vi "View-camera-settings-with-dialog.vi"(8 "error in (no error)":errorcluster, 10 "UI ref. in":refnum<data-value>, 11 "Data ref. in":refnum<data-value>) -> (0 "error out":errorcluster, 3 "Data ref.":refnum<data-value>)   [LabVIEW 2013, in "CameraVision.lvlib" / "CV-Main.lvclass"]
uses:
  CV-Main.lvclass
  UI/CV-UI.lvclass
  CV-Main.lvclass/CV-Main.ctl
  Configuration/CV-Configuration.lvclass/CV-Configuration.ctl
  UI/CV-UI.lvclass/CV-UI.ctl
  Hardware/Camera/Camera.lvclass
  Read Config params.vi
  Configuration/Read Camera array.vi
  Configuration/Read Camport array.vi
  Configuration/Read Framegrabber board.vi
  UI/Read Camera.vi
  Configuration/CV-Configuration.lvclass
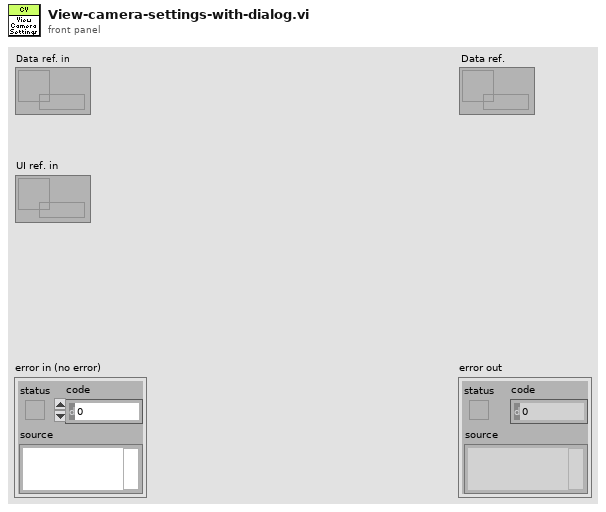
[diagram p1: front panel]
types:
  T1 = typedef "CameraVision.lvlib/CV-UI.lvclass/Camera-selector.ctl" = enum16{"Camera 1", "Camera 2"}
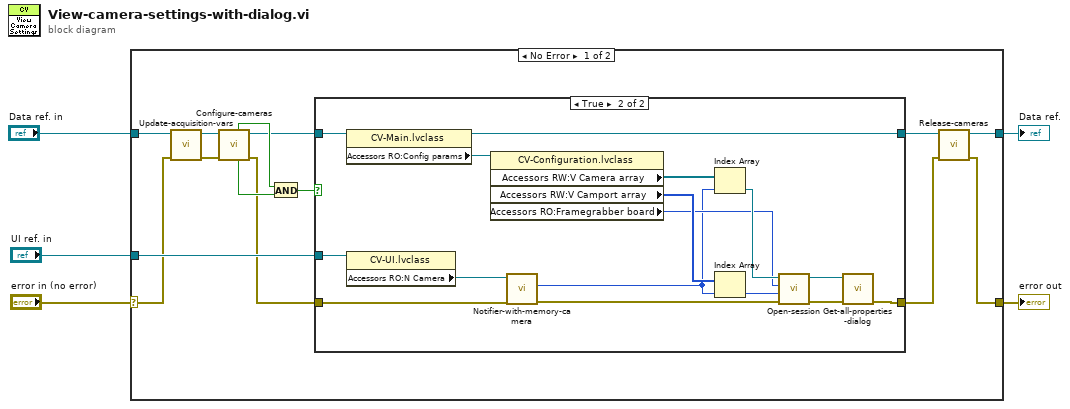
[diagram p0: block diagram]
diagram:
  n1 = case shown="No Error" "error in (no error)" {
    selector: "error in (no error)" -> [w10 w39]
    tunnel: [w9 w39] -> w4
    tunnel: [w6 w38] -> w2
    tunnel: "Data ref. in" -> [w14 w38]
    tunnel: "UI ref. in" -> [w19 _]
    frame No Error {
      n2 = call "Update-acquisition-vars.vi"("error in"=w10, "Data ref. in"=w14) -> ("error IO"=w16:errorcluster, "Data ref."=w15:refnum<data-value>)  [unwired: 6 in, 2 out]
      n3 = call "Configure-cameras.vi"("error in"=w16, "Data ref. in"=w15) -> ("error IO"=w11:errorcluster, "Data ref."=w13:refnum<data-value>, "Initialized?"=w18:bool, "Succes?"=w17:bool)  [unwired: 6 in]
      n4 = And(x=w17, y=w18) -> (x .and. y?=w12:bool)
      n5 = case shown="True" w12 {
        tunnel: [w21 w37] -> w7
        tunnel: w19 -> [_ w35]
        tunnel: w11 -> [w20 w32]
        tunnel: [w20 w24] -> w8
        tunnel: w13 -> [w21 w22]
        frame False {
        }
        frame True {
          n6 = property class="CV-Main.lvclass"(reference=w22) -> (reference out=w37:refnum<data-value>, "Accessors RO:Config params"=w36:refnum<data-value>)  [unwired: 1 in, 1 out]
          n7 = property class="CV-UI.lvclass"(reference=w35) -> ("Accessors RO:N Camera"=w34:refnum<notifier>)  [unwired: 1 in, 2 out]
          n8 = property class="CV-Configuration.lvclass"(reference=w36) -> ("Accessors RW:V Camera array"=w33:refnum<class "Camera.lvclass">[], "Accessors RW:V Camport array"=w27:u32[], "Accessors RO:Framegrabber board"=w26:i32)  [unwired: 1 in, 2 out]
          n9 = call "Notifier-with-memory-camera.vi"("error in"=w32, "Notifier in"=w34) -> ("error IO"=w29:errorcluster, "Notification"=w23:T1)  [unwired: 8 in]
          n10 = Index Array(array=w33, index=w23) -> (element=w30:refnum<class "Camera.lvclass">)
          n11 = Index Array(array=w27, index=w23) -> (element=w25:u32)
          n12 = call-dynamic "Open-session.vi"("error in (no error)"=w29, "Camport"=w25, "Framegrabber board"=w26, "Camera in"=w30) -> ("error out"=w28:errorcluster, "Camera out"=w31:refnum<class "Camera.lvclass">)  [unwired: 5 in, 1 out]
          n13 = call-dynamic "Get-all-properties-dialog.vi"("error in (no error)"=w28, "Camera in"=w31) -> ("error out"=w24:errorcluster)  [unwired: 8 in, 1 out]
        }
      }
      n14 = call "Release-cameras.vi"("error in"=w8, "Data ref. in"=w7) -> ("error IO"=w9:errorcluster, "Data ref."=w6:refnum<data-value>)  [unwired: 8 in]
    }
    frame Error {
    }
  }
  "error out" <- w4
  "Data ref." <- w2
